vi "capbr single measurement.vi"(0 "error in":errorcluster {"code" format="%.0x"}) -> (1 "Voltage":dbl format="%_9f", 2 "Loss":dbl format="%_9f", 3 "Capacitance":dbl format="%_9f", 4 "error out":errorcluster {"code" format="%.0x"})   [LabVIEW 2016, in "AH2500A.lvclass"]
doc: "Use this template to parse data acquired from an instrument attached to your computer through a GPIB, serial, or other port and write the data to a file. Note: VIs created from this template will have automatic error handling enabled by default."
uses:
  SMOs/AH2500A/AH2500A.lvclass
  Instance           1 32Saved   capbr single measurement .vi
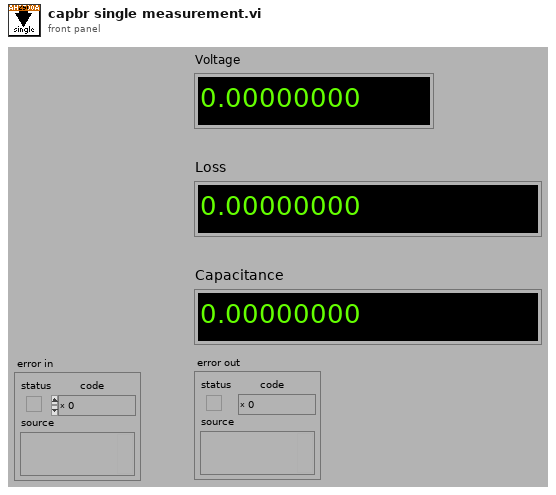
[diagram p1: front panel]
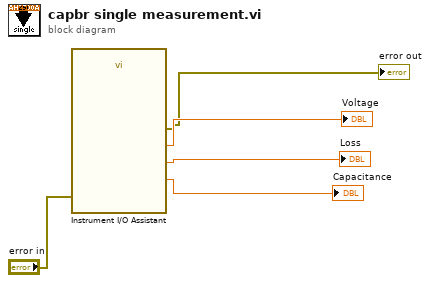
[diagram p0: block diagram]
diagram:
  n1 = call "Instrument I/O Assistant"("error in"="error in") -> ("error out"=→"error out":errorcluster, "Voltage"=→"Voltage":dbl, "Loss"=→"Loss":dbl, "Capacitance"=→"Capacitance":dbl)  [unwired: 7 in]
